vi "FPGA Output Read.vi"(8 "error in (no error)":errorcluster, 11 "RT data in":T1) -> (0 "error out":errorcluster, 3 "RT data out":T1)   [LabVIEW 2011, in "Engine Sim RT.lvlib"]
uses:
  Engine Sim RT.lvlib
  TypeDefs/RT Data Cluster.ctl
  Shared/Channel Descriptors.ctl
  Shared/FPGA Write Descriptor.ctl
  Shared/InputChannelTypes.ctl
  <vilib>/rvi/DataTransferAndStorage/Container/Common/niFpgaDataTypeControl.ctl
  Shared/FPGA Read Descriptor.ctl
  Shared/OutputChannelTypes.ctl
  Shared/Status Chan Descriptor.ctl
  Shared/DataReplayVoltageConfig.ctl
  <userlib>/_FPGA Interface Advanced Tools/FPGA Interface Wrapper/NiFPGA Read - U64.vi
  <userlib>/_FPGA Interface Advanced Tools/FPGA Interface Wrapper/NiFPGA Read - U32.vi
  <vilib>/Utility/error.llb/Error Cluster From Error Code.vi
  <userlib>/_FPGA Interface Advanced Tools/FPGA Interface Wrapper/FPGA Interface Wrapper.lvlib
  Engine Simulation Shared.lvlib
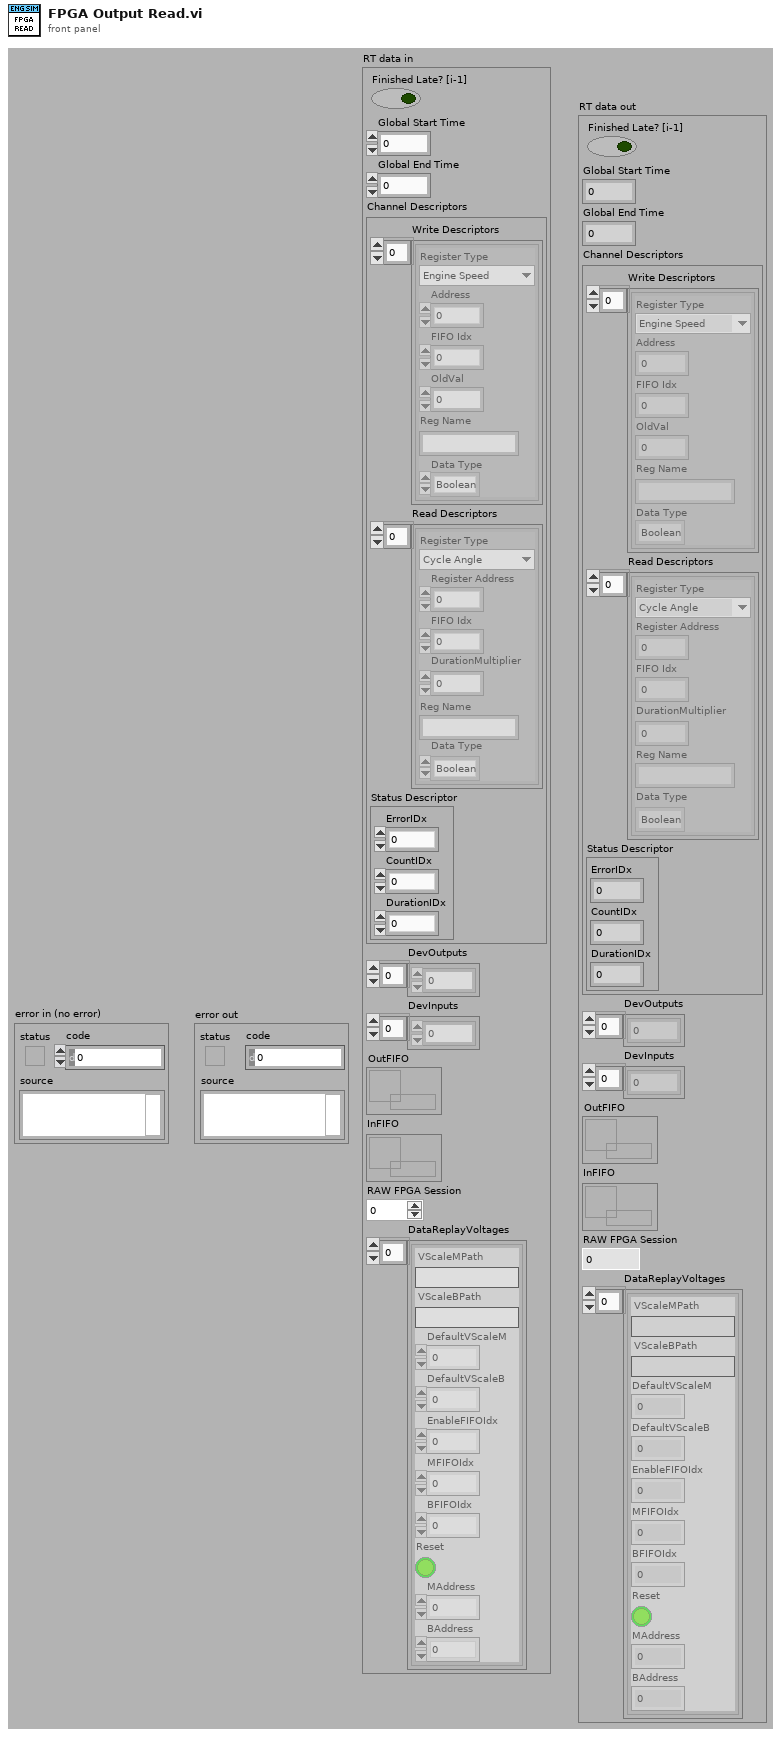
[diagram p1: front panel]
types:
  T1 = typedef "Engine Sim RT.lvlib/RT Data Cluster.ctl" = cluster{"Finished Late? [i-1]":bool, "Global Start Time":i64, "Global End Time":i64, "Channel Descriptors":T2, "DevOutputs":dbl[], "DevInputs":dbl[], "OutFIFO":refnum<k33>, "InFIFO":refnum<k33>, "RAW FPGA Session":u32, "DataReplayVoltages":T9[]}
  T2 = typedef "Engine Simulation Shared.lvlib/Channel Descriptors.ctl" = cluster{"Write Descriptors":T3[], "Read Descriptors":T6[], "Status Descriptor":T8}
  T3 = typedef "Engine Simulation Shared.lvlib/FPGA Write Descriptor.ctl" = cluster{"Register Type":T4, "Address":u32, "FIFO Idx":i32, "OldVal":dbl, "Reg Name":string, "Data Type":T5}
  T4 = typedef "Engine Simulation Shared.lvlib/InputChannelTypes.ctl" = enum16{"Engine Speed", "Offset"}
  T5 = typedef "niFpgaDataTypeControl.ctl" = enum32{"Boolean", "I8", "I16", "I32", "I64", "U8", "U16", "U32", "U64", "FXP", "CustomControl"}
  T6 = typedef "Engine Simulation Shared.lvlib/FPGA Read Descriptor.ctl" = cluster{"Register Type":T7, "Register Address":u32, "FIFO Idx":i32, "DurationMultiplier":dbl, "Reg Name":string, "Data Type":T5}
  T7 = typedef "Engine Simulation Shared.lvlib/OutputChannelTypes.ctl" = enum16{"Cycle Angle", "Crank Angle", "Time Duration", "Angle Duration", "Start Angle", "End Angle"}
  T8 = typedef "Engine Simulation Shared.lvlib/Status Chan Descriptor.ctl" = cluster{"ErrorIDx":i32, "CountIDx":i32, "DurationIDx":i32}
  T9 = typedef "Engine Simulation Shared.lvlib/DataReplayVoltageConfig.ctl" = cluster{"VScaleMPath":string, "VScaleBPath":string, "DefaultVScaleM":u32, "DefaultVScaleB":i32, "EnableFIFOIdx":i32, "MFIFOIdx":i32, "BFIFOIdx":i32, "Reset":bool, "MAddress":u32, "BAddress":u32}
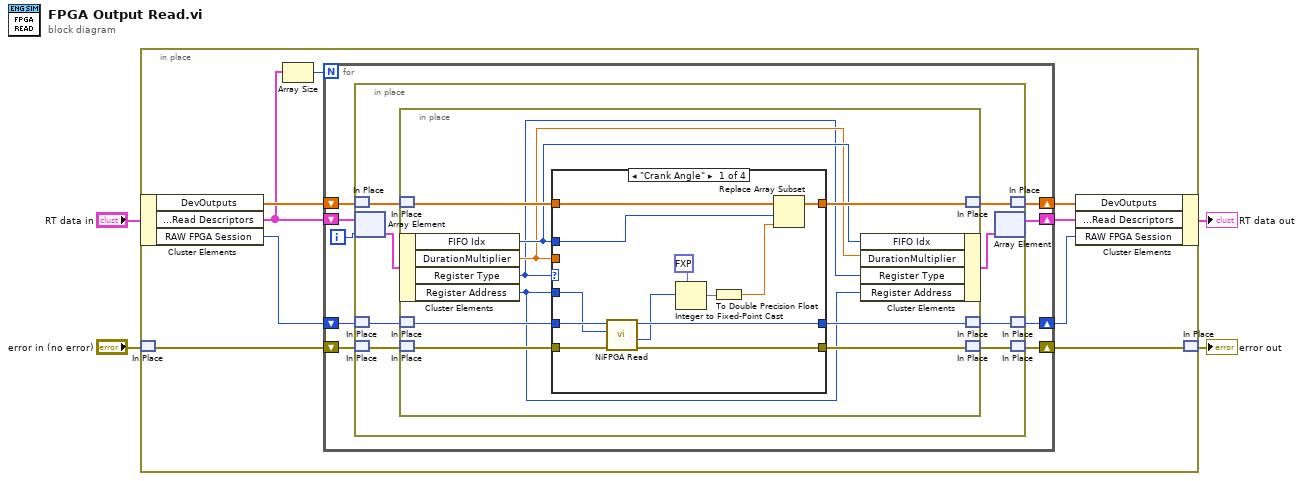
[diagram p0: block diagram]
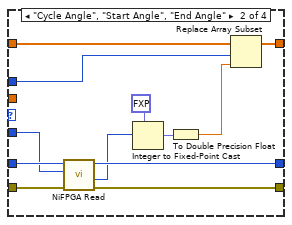
[diagram p2: hidden frame]
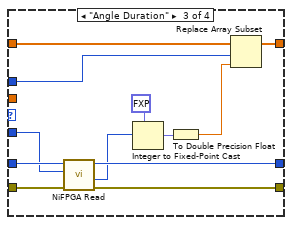
[diagram p3: hidden frame]
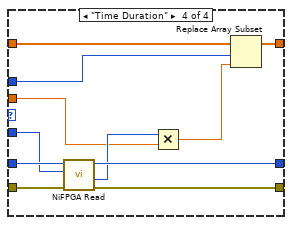
[diagram p4: hidden frame]
diagram:
  n1 = in-place {
    n2 = in-place-cluster #1("RT data in") -> ("DevOutputs"=w9:dbl[], "Channel Descriptors.Read Descriptors"=w6:T6[], "RAW FPGA Session"=w11:u32)
    n3 = in-place-match #2("error in (no error)") -> (w13:errorcluster)
    n4 = Array Size(array=w6) -> (size(s)=w7:i32)
    n5 = for {
      N: w7 -> [_]
      shift-right: [w21] -> w12
      shift-left: w13 -> [w22]
      shift-right: [w19] -> w10
      shift-left: w11 -> [w20]
      shift-right: [w17] -> w8
      shift-left: w9 -> [w18]
      shift-right: [w14] -> w5
      shift-left: w6 -> [w16]
      i -> [w15]
      n6 = in-place {
        n7 = in-place-match #3(w18) -> (w26:dbl[])
        n8 = in-place-array #4(w16, w15) -> (w24:T6)
        n9 = in-place-match #5(w20) -> (w28:u32)
        n10 = in-place-match #6(w22) -> (w30:errorcluster)
        n11 = in-place {
          n12 = in-place-match #7(w26) -> (w37:dbl[])
          n13 = in-place-cluster #8(w24) -> ("FIFO Idx"=w34:i32, "DurationMultiplier"=w33:dbl, "Register Type"=w32:T7, "Register Address"=w31:u32)
          n14 = in-place-match #9(w28) -> (w38:u32)
          n15 = in-place-match #10(w30) -> (w40:errorcluster)
          n16 = case shown="\"Crank Angle\"" w32 {
            tunnel: w31 -> [w41 w53 w65 w78]
            tunnel: w38 -> [w48 w62 w74 w85]
            tunnel: w40 -> [w50 w64 w76 w87]
            tunnel: [w49 w63 w75 w86] -> w39
            tunnel: [w45 w60 w72 w83] -> w36
            tunnel: w37 -> [w44 w59 w71 w82]
            tunnel: [w47 w61 w73 w84] -> w35
            tunnel: w34 -> [w42 w58 w70 w81]
            tunnel: w33 -> [_ _ _ w77]
            frame "Crank Angle" {
              n17 = call-poly <userlib>:"NiFPGA Read.vi"("error in (no error)"=w50, "Indicator"=w41, "Session"=w48) -> ("error out"=w49:errorcluster, "Value"=w46:u64, "Session Out"=w47:u32)  [unwired: 6 in]
              n18 = Integer to Fixed-Point Cast(fixed-point type=fxp<+,60,9> 0.0, integer=w46) -> (fixed-point=w51:fxp<+,60,9>)
              n19 = To Double Precision Float(number=w51) -> (double precision float=w43:dbl)
              n20 = Replace Array Subset(array=w44, new element=w43, index=w42) -> (w45:dbl[])
            }
            frame "Cycle Angle", "Start Angle", "End Angle" {
              n21 = call-poly <userlib>:"NiFPGA Read.vi"("error in (no error)"=w64, "Indicator"=w53, "Session"=w62) -> ("error out"=w63:errorcluster, "Value"=w55:u64, "Session Out"=w61:u32)  [unwired: 6 in]
              n22 = Integer to Fixed-Point Cast(fixed-point type=fxp<+,61,10> 0.0, integer=w55) -> (fixed-point=w56:fxp<+,61,10>)
              n23 = To Double Precision Float(number=w56) -> (double precision float=w54:dbl)
              n24 = Replace Array Subset(array=w59, new element=w54, index=w58) -> (w60:dbl[])
            }
            frame "Angle Duration" {
              n25 = call-poly <userlib>:"NiFPGA Read.vi"("error in (no error)"=w76, "Indicator"=w65, "Session"=w74) -> ("error out"=w75:errorcluster, "Value"=w67:u64, "Session Out"=w73:u32)  [unwired: 6 in]
              n26 = Integer to Fixed-Point Cast(fixed-point type=fxp<+/-,62,11> 0.0, integer=w67) -> (fixed-point=w68:fxp<+/-,62,11>)
              n27 = To Double Precision Float(number=w68) -> (double precision float=w66:dbl)
              n28 = Replace Array Subset(array=w71, new element=w66, index=w70) -> (w72:dbl[])
            }
            frame "Time Duration" {
              n29 = call-poly <userlib>:"NiFPGA Read.vi"("error in (no error)"=w87, "Indicator"=w78, "Session"=w85) -> ("error out"=w86:errorcluster, "Value"=w80:u32, "Session Out"=w84:u32)  [unwired: 6 in]
              n30 = Multiply(x=w80, y=w77) -> (x*y=w79:dbl)
              n31 = Replace Array Subset(array=w82, new element=w79, index=w81) -> (w83:dbl[])
            }
          }
          n32 = in-place-cluster #8("FIFO Idx"=w34, "DurationMultiplier"=w33, "Register Type"=w32, "Register Address"=w31) -> (w23:T6)
          n33 = in-place-match #7(w36) -> (w25:dbl[])
          n34 = in-place-match #9(w35) -> (w27:u32)
          n35 = in-place-match #10(w39) -> (w29:errorcluster)
        }
        n36 = in-place-array #4(w23) -> (w14:T6[])  [unwired: 1 out]
        n37 = in-place-match #3(w25) -> (w17:dbl[])
        n38 = in-place-match #5(w27) -> (w19:u32)
        n39 = in-place-match #6(w29) -> (w21:errorcluster)
      }
    }
    n40 = in-place-cluster #1("DevOutputs"=w8, "Channel Descriptors.Read Descriptors"=w5, "RAW FPGA Session"=w10) -> (→"RT data out":T1)
    n41 = in-place-match #2(w12) -> (→"error out":errorcluster)
  }
